vi "Update Casing Style.vi"(11 "Input Name":string) -> (2 "snake_case":string, 3 "PascalCase":string)   [LabVIEW 2021, in "Plugin Generator.lvlib"]
uses:
  Plugin Generator.lvlib
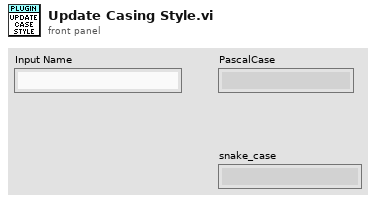
[diagram p1: front panel]
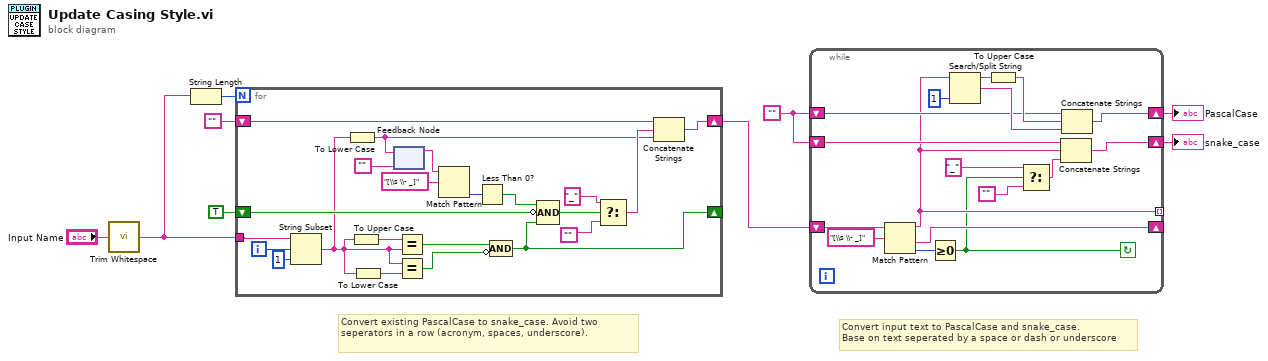
[diagram p0: block diagram]
diagram:
  w9 = ""
  # "Convert existing PascalCase to snake_case. Avoid two seperators in a row (acronym, spaces, underscore)."
  # "Convert input text to PascalCase and snake_case.\nBase on text seperated by a space or dash or underscore"
  n1 = call <vilib>:"Trim Whitespace.vi"("string"="Input Name") -> ("trimmed string"=w2:string)  [unwired: 1 in]
  n2 = String Length(string=w2) -> (length=w4:i32)
  n3 = for {
    N: w4 -> [_]
    tunnel: w2 -> [w31]
    shift-right: [w21] -> w1
    shift-left: "" -> [w28]
    shift-right: [w17] -> _
    shift-left: TRUE -> [w20]
    i -> [w30]
    n4 = String Subset(string=w31, offset (0)=w30, length (rest)=1 ("length (rest)")) -> (substring=w19:string)
    n5 = To Lower Case(string=w19) -> (all lower case string=w15:string)
    n6 = To Upper Case(1:w19) -> (0:w27:string)
    n7 = To Lower Case(string=w19) -> (all lower case string=w24:string)
    n8 = feedback-in #1(w15) -> ()
    n9 = feedback #1("") -> (w12:string)
    n10 = Equal?(x=w27, y=w19) -> (x = y?=w23:bool)
    n11 = Equal?(x=w19, y=w24) -> (x = y?=w22:bool)
    n12 = Match Pattern(string=w12, regular expression="[\\s \\- _]") -> (offset past match=w11:i32)  [unwired: 1 in, 3 out]
    n13 = Less Than 0?(x=w11) -> (x < 0?=w10:bool)
    n14 = Compound Arithmetic op=AND(w23, invert w22) -> (w17:bool)
    n15 = Compound Arithmetic op=AND(w10, invert w20, w17) -> (w16:bool)
    n16 = Select(t="_", s=w16, f="") -> (s? t:f=w18:string)
    n17 = Concatenate Strings(w28, w18, w15) -> (w21:string)
  }
  n18 = while {
    tunnel: [w37] -> _ mode=indexing
    shift-right: [w45] -> _
    shift-left: w1 -> [w48]
    shift-right: [w33] -> w8
    shift-left: w9 -> [w38]
    shift-right: [w39] -> w7
    shift-left: w9 -> [w40]
    stop <- w35 continue-if-true
    n19 = Match Pattern(string=w48, regular expression="[\\s \\- _]") -> (before substring=w37:string, after substring=w45:string, offset past match=w46:i32)  [unwired: 1 in, 1 out]
    n20 = Greater Or Equal To 0?(x=w46) -> (x >= 0?=w35:bool)
    n21 = Search/Split String(string=w37, offset (0)=1) -> (substring before match=w43:string, match + rest of string=w41:string)  [unwired: 1 in, 1 out]
    n22 = To Upper Case(1:w43) -> (0:w42:string)
    n23 = Select(t="_", s=w35, f="") -> (s? t:f=w36:string)
    n24 = Concatenate Strings(w38, w37, w36) -> (w33:string)
    n25 = Concatenate Strings(w40, w42, w41) -> (w39:string)
  }
  "snake_case" <- w8
  "PascalCase" <- w7
